vi "Restore Modal.vi"   [LabVIEW 2020, in "Conditum-Tools.lvlib"]
uses:
  Conditum-Tools.lvlib
types:
  T1 = enum32{"Invalid", "Default", "Floating", "Floating/Auto-Hide", "Modal"}
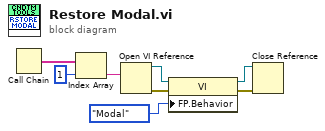
[diagram p0: block diagram]
diagram:
  n1 = Call Chain() -> (call chain=w8:string[])
  n2 = Index Array(array=w8, index=1) -> (element=w7:string)
  n3 = Open VI Reference(vi path=w7) -> (vi reference=w1:refnum<vi>, error out=w2:errorcluster)  [unwired: 5 in]
  n4 = property class="VI"(reference=w1, error in=w2, "FP.Behavior"=T1."Modal" ("Front Panel Window:Behavior")) -> (reference out=w5:refnum<vi>, error out=w6:errorcluster)
  n5 = Close Reference(reference=w5, error in (no error)=w6) -> ()  [unwired: 1 out]
